vi "Connect.vi"(8 "error in (no error)":errorcluster, 11 "reference in":refnum<class "NS slave.lvclass">) -> (0 "error out":errorcluster, 3 "reference out":refnum<class "NS slave.lvclass">)   [LabVIEW 2019, in "CommandResponse communication.lvlib" / "NS slave.lvclass"]
doc: "Connects to Master device and established network streams communication"
uses:
  NS slave.lvclass
  C:/Barkhausen mmWave radar/Development/LV/Barkhausen mmWave hardware control/Host/Intertarget communication/CR slave_class/CR slave.lvclass
  ITC command.ctl
  ITC response.ctl
  CommandResponse communication.lvlib
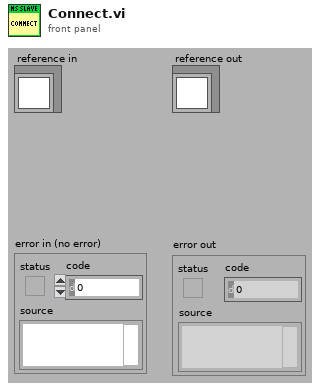
[diagram p1: front panel]
types:
  T1 = typedef "CommandResponse communication.lvlib/ITC response.ctl" = cluster{"status":string, "reponse":string, "data":variant}
  T2 = typedef "CommandResponse communication.lvlib/ITC command.ctl" = cluster{"message":string, "parameters":string, "data":variant}
  T3 = typedef "CommandResponse communication.lvlib/NS slave.lvclass/ObjectAttributes.ctl" = cluster{"connected":bool, "stop":bool, "ID":string, "command rd":refnum<k21>, "response wr":refnum<k21>, "data wr":refnum<k21>}
  T4 = typedef "CommandResponse communication.lvlib/NS slave.lvclass/ObjectAttributesRef.ctl" = refnum<data-value>
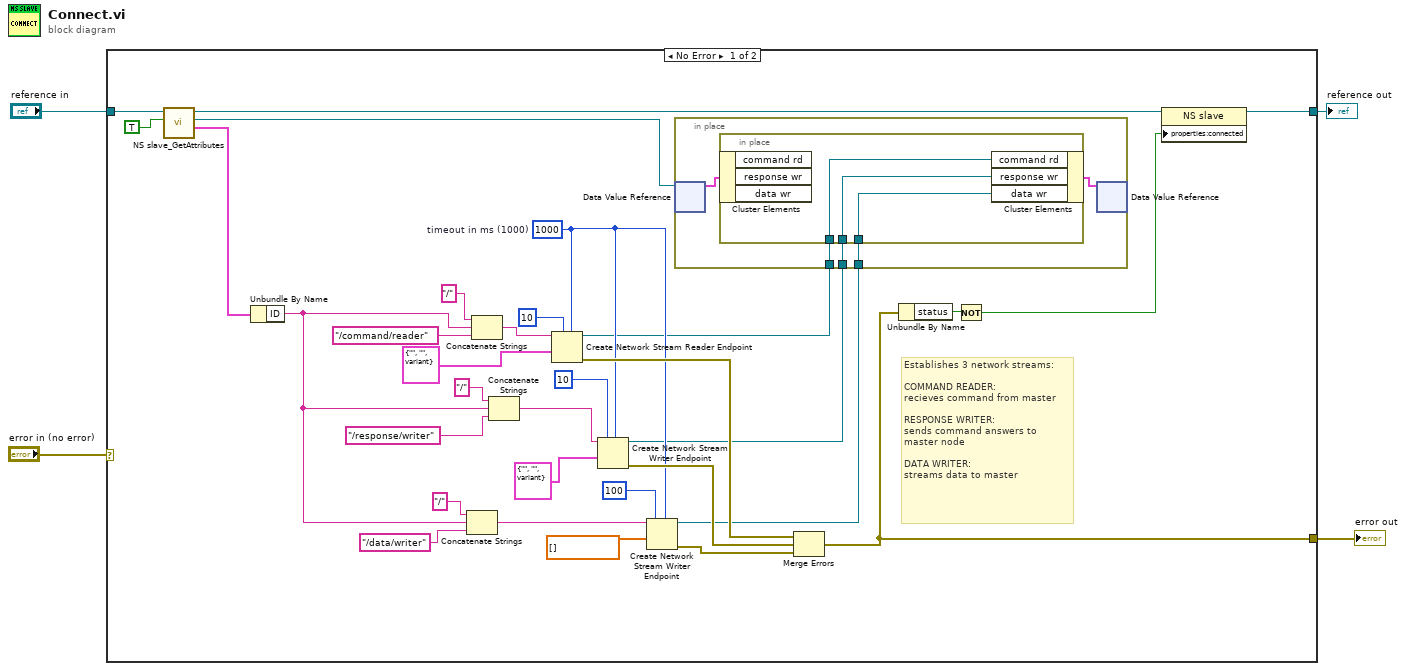
[diagram p0: block diagram]
diagram:
  n1 = case shown="No Error" "error in (no error)" {
    selector: "error in (no error)" -> [_ w46]
    tunnel: [w6 w46] -> w3
    tunnel: [w8 w45] -> w1
    tunnel: "reference in" -> [w35 w45]
    frame No Error {
      w23 = 1000  # timeout in ms (1000)
      # "Establishes 3 network streams:\n\nCOMMAND READER:\nrecieves command from master\n\nRESPONSE WRITER:\nsends command answers to\nmaster node\n\nDATA WRITER:\nstreams data to master"
      n2 = call "NS slave_GetAttributes.vi"("return data? (T)"=TRUE, "reference in"=w35) -> ("attributes"=w18:T3, "attributes ref"=w33:T4, "reference out"=w36:refnum<class "NS slave.lvclass">)  [unwired: 6 in, 1 out]
      n3 = Unbundle By Name(w18) -> ("ID"=w11:string)
      n4 = Concatenate Strings("/" ("string"), w11, "/data/writer" ("reader url")) -> (w9:string)
      n5 = Concatenate Strings("/" ("string"), w11, "/command/reader" ("reader url")) -> (w17:string)
      n6 = Concatenate Strings("/" ("string"), w11, "/response/writer" ("reader url")) -> (w13:string)
      n7 = Create Network Stream Reader Endpoint(5:w23, 7:10 ("writer buffer size"), 9:T2 {"message"="", "parameters"="", "data"=variant} ("command"), 11:w17) -> (0:w29:errorcluster, 3:w21:refnum<k21>)  [unwired: 3 in]
      n8 = Create Network Stream Writer Endpoint(5:w23, 7:10 ("reader buffer size"), 9:T1 {"status"="", "reponse"="", "data"=variant(cluster{"Boolean Round":bool, "code":i32, "source":string} {"Boolean Round"=FALSE, "code"=0, "source"=""})} ("ITC response"), 11:w13) -> (0:w27:errorcluster, 3:w20:refnum<k21>)  [unwired: 3 in]
      n9 = Create Network Stream Writer Endpoint(5:w23, 7:100 ("reader buffer size"), 9:cdb[] [] ("data"), 11:w9) -> (0:w22:errorcluster, 3:w19:refnum<k21>)  [unwired: 3 in]
      n10 = in-place {
        in-place-border: w21 -> [w39]
        in-place-border: w20 -> [w38]
        in-place-border: w19 -> [w37]
        n11 = in-place-dvr #1(w33) -> (w41:T3)  [unwired: 1 out]
        n12 = in-place {
          in-place-border: w39 -> [w44]
          in-place-border: w38 -> [w43]
          in-place-border: w37 -> [w42]
          n13 = in-place-cluster #2(w41) -> ()  [unwired: 3 out]
          n14 = in-place-cluster #2("command rd"=w44, "response wr"=w43, "data wr"=w42) -> (w40:T3)
        }
        n15 = in-place-dvr #1(w40) -> ()  [unwired: 2 out]
      }
      n16 = Merge Errors(w29, w27, w22) -> (w6:errorcluster)
      n17 = Unbundle By Name(w6) -> ("status"=w7:bool)
      n18 = Not(x=w7) -> (.not. x?=w5:bool)
      n19 = property class="NS slave"(reference=w36, "properties:connected"=w5) -> (reference out=w8:refnum<class "NS slave.lvclass">)  [unwired: 1 in, 1 out]
    }
    frame Error {
    }
  }
  "error out" <- w3
  "reference out" <- w1
